vi "Test Work Dispatcher Forward Message When Adding Worker.vi"(8 "error in (no error)":errorcluster, 11 "Work Dispatcher Test in":refnum<class "Work Dispatcher Test.lvclass">=refnum) -> (0 "error out":errorcluster, 3 "Work Dispatcher Test out":refnum<class "Work Dispatcher Test.lvclass">)   [LabVIEW 2020, in "Work Dispatcher Test.lvclass"]
uses:
  Work Dispatcher Test.lvclass
  <vilib>/Astemes/Triarc Framework/Process/Process.lvclass
  Processes/Work Dispatcher/Work Dispatcher.lvclass
  Test Doubles/Mock Job Handler/Mock Job Handler.lvclass
  <vilib>/Astemes/LUnit/Test Case.lvclass
  C:/Program Files (x86)/National Instruments/LabVIEW 2020/vi.lib/Astemes/Triarc Framework/Process/Process.lvclass
  C:/Program Files (x86)/National Instruments/LabVIEW 2020/vi.lib/Astemes/Triarc Framework/Base/Base.lvclass
  C:/Program Files (x86)/National Instruments/LabVIEW 2020/vi.lib/Astemes/Triarc Framework/Error Handler Interface/Error Handler Interface.lvclass
  C:/Program Files (x86)/National Instruments/LabVIEW 2020/vi.lib/Astemes/Triarc Framework/Logging/Logging.lvclass
  C:/git/astemes-triarc-examples/source/Coffee Shop/Processes/Work Dispatcher/Work Dispatcher.lvclass
  C:/git/astemes-triarc-examples/source/Coffee Shop/Processes/People/Process Job/Job Handler.lvclass
  C:/Program Files (x86)/National Instruments/LabVIEW 2020/vi.lib/Astemes/Triarc Framework/Helper Loop/Helper Loop.lvclass
  C:/Program Files (x86)/National Instruments/LabVIEW 2020/vi.lib/Astemes/LUnit/Test Case.lvclass
  C:/Program Files (x86)/National Instruments/LabVIEW 2020/vi.lib/Astemes/LUnit/LUnit Runnable.lvclass
  C:/git/astemes-triarc-examples/source/Coffee Shop/Tests/Test Doubles/Mock Job Handler/Mock Job Handler.lvclass
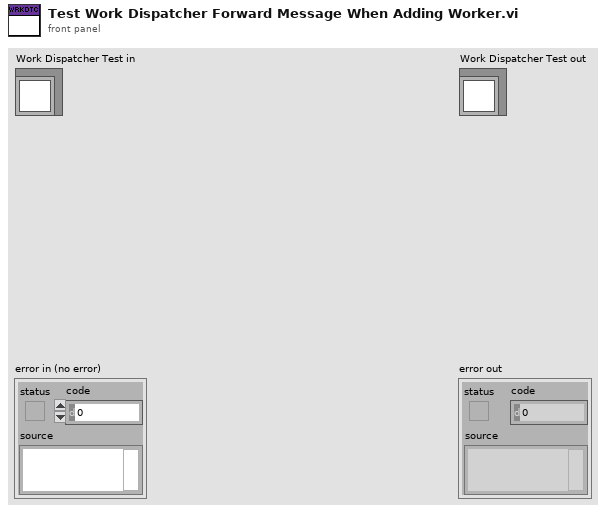
[diagram p1: front panel]
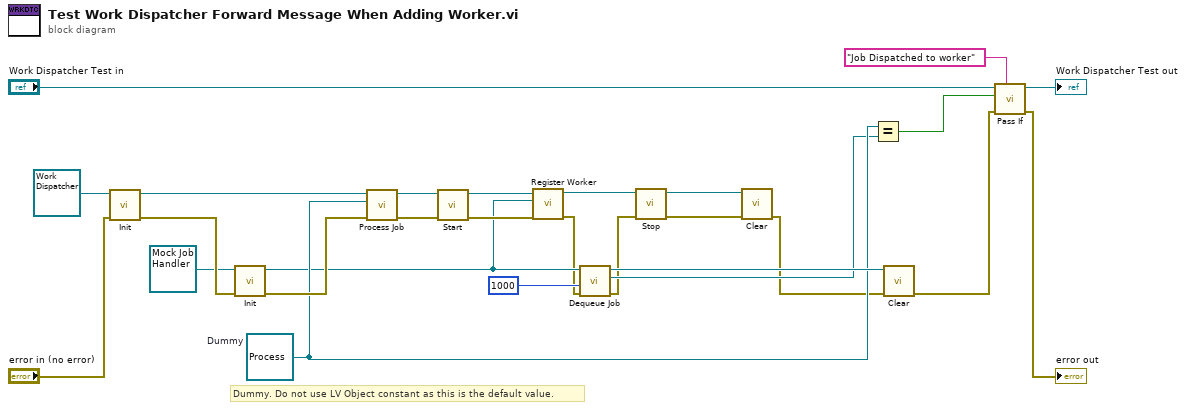
[diagram p0: block diagram]
diagram:
  w14 = refnum<class "Process.lvclass"> refnum  # Dummy
  # "Dummy. Do not use LV Object constant as this is the default value."
  n1 = call-dynamic "Init.vi"("error in (no error)"="error in (no error)", "Process In"=refnum<class "Work Dispatcher.lvclass"> refnum ("Work Dispatcher.lvclass")) -> ("error out"=w24:errorcluster, "Process Out"=w25:refnum<class "Work Dispatcher.lvclass">)  [unwired: 8 in]
  n2 = call-dynamic "Init.vi"("error in (no error)"=w24, "Mock Job Handler In"=refnum<class "Mock Job Handler.lvclass"> refnum ("Mock Worker In")) -> ("error out"=w18:errorcluster, "Mock Job Handler Out"=w5:refnum<class "Mock Job Handler.lvclass">)  [unwired: 8 in]
  n3 = call-dynamic "Process Job.vi"("error in (no error)"=w18, "Task"=w14, "Work Dispatcher In"=w25) -> ("error out"=w16:errorcluster, "Work Dispatcher Out"=w17:refnum<class "Work Dispatcher.lvclass">)  [unwired: 7 in]
  n4 = call <vilib>:"Start.vi"("error in (no error)"=w16, "Process In"=w17) -> ("error out"=w19:errorcluster, "Process Out"=w7:refnum<class "Work Dispatcher.lvclass">)  [unwired: 7 in, 1 out]
  n5 = call-dynamic "Register Worker.vi"("error in (no error)"=w19, "Worker"=w5, "Work Dispatcher In"=w7) -> ("error out"=w3:errorcluster, "Work Dispatcher Out"=w6:refnum<class "Work Dispatcher.lvclass">)  [unwired: 7 in]
  n6 = call "Dequeue Job.vi"("error in (no error)"=w3, "timeout in ms (-1)"=1000, "Mock Job Handler In"=w5) -> ("error out"=w2:errorcluster, "element"=w13:refnum<class>, "Mock Job Handler Out"=w20:refnum<class "Mock Job Handler.lvclass">)  [unwired: 5 in, 1 out]
  n7 = call <vilib>:"Stop.vi"("error in (no error)"=w2, "Process In"=w6) -> ("error out"=w22:errorcluster, "Process Out"=w23:refnum<class "Work Dispatcher.lvclass">)  [unwired: 7 in, 1 out]
  n8 = call-dynamic "Clear.vi"("error in (no error)"=w22, "Process In"=w23) -> ("error out"=w1:errorcluster)  [unwired: 9 in]
  n9 = Equal?(x=w14, y=w13) -> (x = y?=w10:bool)
  n10 = call-dynamic "Clear.vi"("error in (no error)"=w1, "Mock Job Handler In"=w20) -> ("error out"=w9:errorcluster)  [unwired: 9 in]
  n11 = call <vilib>:"Pass If.vi"("Description"="Job Dispatched to worker", "error in (no error)"=w9, "Pass?"=w10, "LUnit Test Case In"="Work Dispatcher Test in") -> ("error out"=→"error out":errorcluster, "LUnit Test Case Out"=→"Work Dispatcher Test out":refnum<class "Test Case.lvclass">)  [unwired: 6 in]
